vi "시간지연.vi"() -> ()   [LabVIEW 2014]
uses:
  <vilib>/Instr/_visa.llb/VISA Configure Serial Port (Instr).vi
panel:
  out "버퍼 읽기":string
  in  "버퍼 쓰기":string
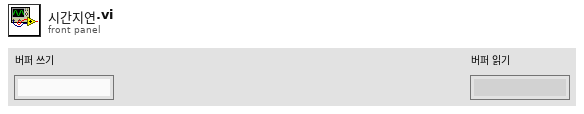
[diagram p1: front panel]
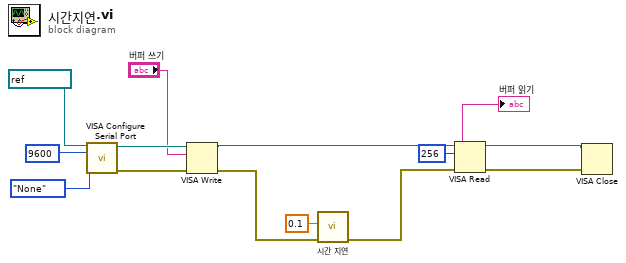
[diagram p0: block diagram]
diagram:
  n1 = call-poly "VISA Configure Serial Port"("VISA resource name"=refnum<visa-resource-name> "COM1", "baud rate (9600)"=u32 9600, "parity (0:none)"=enum16{"None", "Odd", "Even", "Mark", "Space"}."None") -> ("VISA resource name out"=w11:refnum<visa-resource-name>, "error out"=w10:errorcluster)  [unwired: 11 in]
  n2 = VISA Write(VISA resource name=w11, write buffer="버퍼 쓰기", error in (no error)=w10) -> (VISA resource name out=w3:refnum<visa-resource-name>, error out=w2:errorcluster)  [unwired: 1 out]
  n3 = call "시간 지연"("error in (no error)"=w2, "Delay Time (s)"=0.1) -> ("error out"=w1:errorcluster)  [unwired: 9 in]
  n4 = VISA Read(VISA resource name=w3, byte count=u32 256 ("바이트 카운트"), error in (no error)=w1) -> (VISA resource name out=w7:refnum<visa-resource-name>, read buffer=→"버퍼 읽기":string, error out=w6:errorcluster)  [unwired: 1 out]
  n5 = VISA Close(VISA resource name=w7, error in (no error)=w6) -> ()  [unwired: 1 out]
